vi "Get Pressure Servo Valve Value.vi"(8 "error in (no error)":errorcluster, 11 "ILC TV Closed Loop Actuator Cylinder in":refnum<class "ILC TV Closed Loop Actuator Cylinder.lvclass">) -> (0 "error out":errorcluster, 2 "Value":dbl format="%.2f", 3 "ILC TV Closed Loop Actuator Cylinder out":refnum<class "ILC TV Closed Loop Actuator Cylinder.lvclass">)   [LabVIEW 2015, in "ILC TV Closed Loop Actuator Cylinder.lvclass"]
uses:
  ILC TV Closed Loop Actuator Cylinder.lvclass
  ILC Actuator Cylinder/ILC Actuator Cylinder.lvclass/ILC Actuator Cylinder.ctl
  ILC Actuator Cylinder/ILC Actuator Cylinder.lvclass
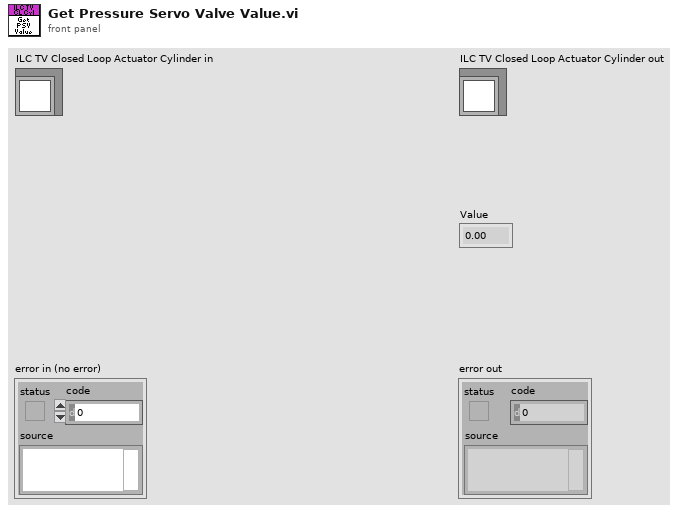
[diagram p1: front panel]
types:
  T1 = typedef "FAMT Typedefs.lvlib/Pressure Servo Valve Settings.ctl" = cluster{"Center Point":dbl[unit], "Area":dbl, "PA to PSI":dbl, "Off Value":dbl}
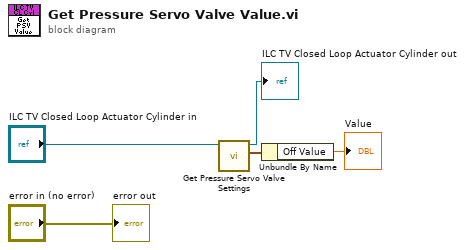
[diagram p0: block diagram]
diagram:
  n1 = call "Get Pressure Servo Valve Settings.vi"("ILC Actuator Cylinder in"="ILC TV Closed Loop Actuator Cylinder in") -> ("Pressure Servo Settings"=w1:T1, "ILC Actuator Cylinder out"=→"ILC TV Closed Loop Actuator Cylinder out":refnum<class "ILC TV Closed Loop Actuator Cylinder.lvclass">)  [unwired: 9 in]
  n2 = Unbundle By Name(w1) -> ("Off Value"=→"Value":dbl)
  "error out" <- "error in (no error)"
